vi "UpdateUserInfo.vi"(8 "error in":errorcluster, 10 "User":T1={"UserName"="", "Password"="", "Role"=enum."Admin"}, 11 "User List":T1[](array[typedef])) -> (0 "error out":errorcluster, 3 "User List":T1[](array[typedef]))   [LabVIEW 2020, in "Login-UI.lvlib" / "PwdMgr.lvclass"]
uses:
  PwdMgr.lvclass
  _Typedef/User-Info.ctl
  _Typedef/User-Role.ctl
  Login-UI.lvlib
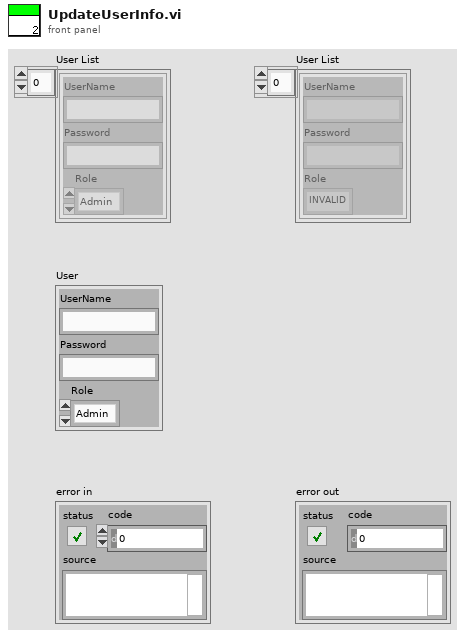
[diagram p1: front panel]
types:
  T1 = typedef "Login-UI.lvlib/User-Info.ctl" = cluster{"UserName":string, "Password":string, "Role":T2}
  T2 = typedef "Login-UI.lvlib/User-Role.ctl" = enum16{"INVALID", "Operator", "Engineer", "Admin", "Anonymous"}
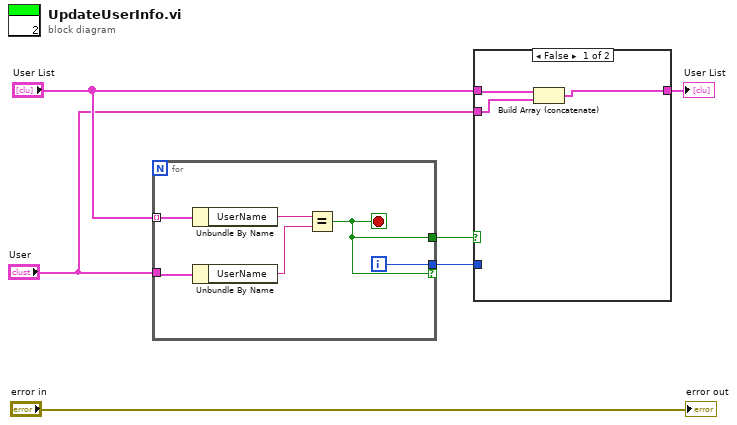
[diagram p0: block diagram]
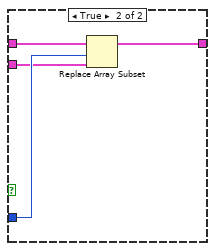
[diagram p2: hidden frame]
diagram:
  n1 = for {
    tunnel: "User List" -> [w12] mode=indexing
    tunnel: "User" -> [w10]
    tunnel: [w8] -> w4 if=w7
    tunnel: [w7] -> w6
    i -> [w8]
    stop <- w7 stop-if-true
    n2 = Unbundle By Name(w12) -> ("UserName"=w11:string)
    n3 = Unbundle By Name(w10) -> ("UserName"=w9:string)
    n4 = Equal?(x=w11, y=w9) -> (x = y?=w7:bool)
  }
  n5 = case shown="False" w6 {
    tunnel: "User List" -> [w15 w19]
    tunnel: w4 -> [_ w17]
    tunnel: [w13 w18] -> w3
    tunnel: "User" -> [w14 w16]
    frame False {
      n6 = Build Array (concatenate)(w15, w14) -> (w13:T1[])
    }
    frame True {
      n7 = Replace Array Subset(array=w19, new element=w16, index=w17) -> (w18:T1[])
    }
  }
  "User List" <- w3
  "error out" <- "error in"
